vi "Link Control References.vi"(8 "error in (no error)":errorcluster, 10 "Control Map":T1[](array[typedef]), 11 "Instruments in":refnum<class "Instruments.lvclass">) -> (0 "error out":errorcluster, 3 "Instruments out":refnum<class "Instruments.lvclass">)   [LabVIEW 2023, in "Instruments.lvlib" / "Instruments.lvclass"]
uses:
  Library/Instruments.lvclass
  Custom Controls/Control Element.ctl
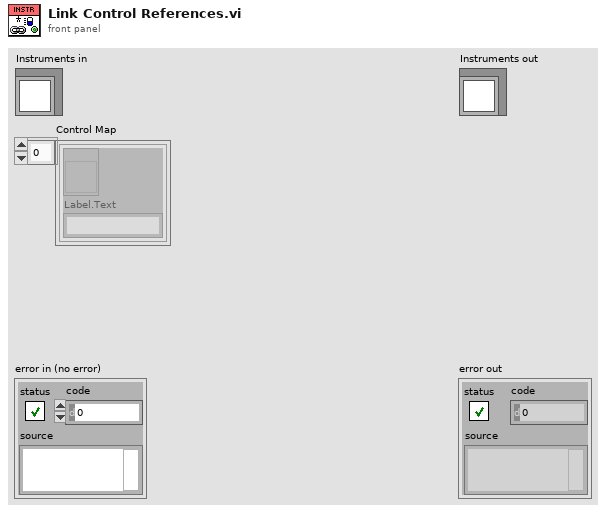
[diagram p1: front panel]
types:
  T1 = typedef "Instruments.lvlib/Instruments.lvclass/Control Element.ctl" = cluster{refnum<vi>, "Label.Text":string}
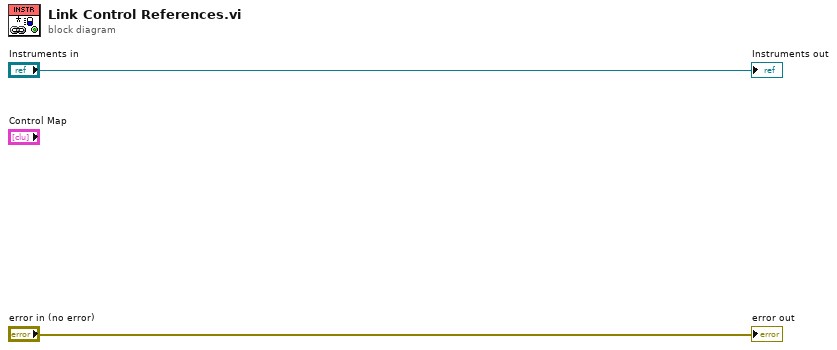
[diagram p0: block diagram]
diagram:
  "error out" <- "error in (no error)"
  "Instruments out" <- "Instruments in"
